vi "getDefaultData.vi"(8 "error in (no error)":errorcluster, 11 "ChannelArray in":refnum<class "ChannelArray.lvclass">) -> (0 "error out":errorcluster, 1 "calibratedValues":dbl[](array[numeric]), 2 "channelAddresses":string[](array[string]), 3 "ChannelArray out":refnum<class "ChannelArray.lvclass">)   [LabVIEW 2009, in "Tools.lvlib" / "DatabaseHelpers.lvlib" / "ChannelArray.lvclass"]
uses:
  ChannelArray.lvclass
  ChannelArray.lvclass/ChannelArray.ctl
  Channel/Channel.lvclass
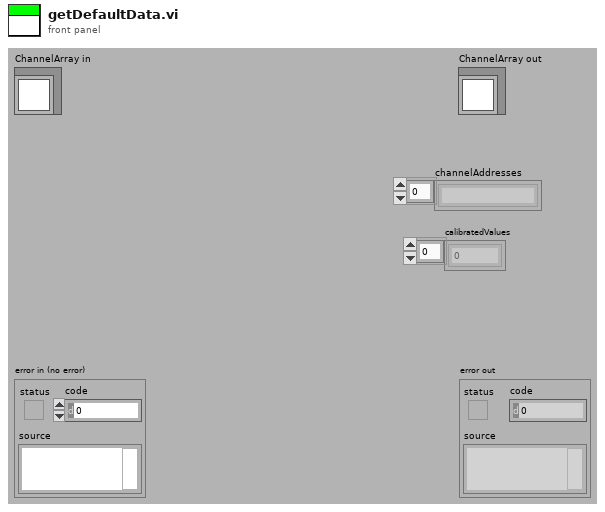
[diagram p1: front panel]
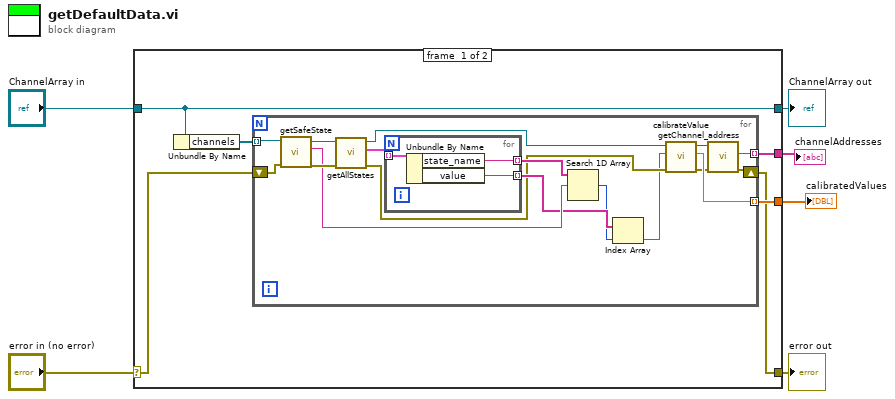
[diagram p0: block diagram]
diagram:
  n1 = case shown="No Error" "error in (no error)" {
    selector: "error in (no error)" -> [w10 w34]
    tunnel: [w8 w34] -> w5
    tunnel: [w12 w33] -> w3
    tunnel: "ChannelArray in" -> [w12 w33]
    tunnel: [w9 _] -> w2
    tunnel: [w7 _] -> w1
    frame #0 {
      n2 = Unbundle By Name(w12) -> ("channels"=w11:refnum<class "Channel.lvclass">[])
      n3 = for {
        tunnel: w11 -> [w29] mode=indexing
        tunnel: [w17] -> w9 mode=indexing
        shift-right: [w13] -> w8
        shift-left: w10 -> [w23]
        tunnel: [w14] -> w7 mode=indexing
        n4 = call "getSafeState.vi"("error in (no error)"=w23, "Channel.lvclass in"=w29) -> ("error out"=w27:errorcluster, "safe_state"=w24:string, "Channel.lvclass out"=w28:refnum<class "Channel.lvclass">)  [unwired: 7 in]
        n5 = call "getAllStates.vi"("error in (no error)"=w27, "Channel.lvclass in"=w28) -> ("error out"=w19:errorcluster, "states"=w26:cluster{"state_name":string, "value":string}[], "Channel.lvclass out"=w20:refnum<class "Channel.lvclass">)  [unwired: 7 in]
        n6 = for {
          tunnel: w26 -> [w32] mode=indexing
          tunnel: [w31] -> w25 mode=indexing
          tunnel: [w30] -> w22 mode=indexing
          n7 = Unbundle By Name(w32) -> ("state_name"=w31:string, "value"=w30:string)
        }
        n8 = Search 1D Array(1D array=w25, element=w24) -> (index of element=w21:i32)  [unwired: 1 in]
        n9 = Index Array(array=w22, index=w21) -> (element=w18:string)
        n10 = call-dynamic "calibrateValue.vi"("error in (no error)"=w19, "value"=w18, "Channel in"=w20) -> ("error out"=w16:errorcluster, "calibratedValue"=w17:dbl, "Channel out"=w15:refnum<class "Channel.lvclass">)  [unwired: 6 in]
        n11 = call "getChannel_address.vi"("error in (no error)"=w16, "Channel.lvclass in"=w15) -> ("error out"=w13:errorcluster, "channel_address"=w14:string)  [unwired: 7 in, 1 out]
      }
    }
    frame #1 {
    }
  }
  "error out" <- w5
  "ChannelArray out" <- w3
  "calibratedValues" <- w2
  "channelAddresses" <- w1
